vi "Periodic Tasks.vi"(8 "error in (no error)":errorcluster) -> ()   [LabVIEW 2015]
doc: "This VI runs in parallel to other tasks. It can contain as many user-defined periodic loops as you need. These can carry out PID or other sorts of timed response."
uses:
  arm/arm.lvclass/arm.ctl
  Robot Global Data.vi
  <vilib>/addons/control/pid/pid.llb/PID (DBL).vi
  <vilib>/Rock Robotics/Network Tables/NT Read Number.vi
  <vilib>/Rock Robotics/Network Tables/NT Write Number.vi
  <vilib>/Rock Robotics/WPI/RobotDrive/WPI_RobotDriveArcadeDrive_Standard(NoSaturation).vi
  <vilib>/addons/control/pid/NI_PID_pid.lvlib
  <vilib>/Analysis/NI_AALPro.lvlib
  shooter/shooter.lvclass
  <vilib>/Analysis/coordinate.llb/2D Cartesian Coordinate Shift (Scalar).vi
  <vilib>/Rock Robotics/Network Tables/NT Read String.vi
  <vilib>/Analysis/coordinate.llb/2D Cartesian Coordinate Shift (Array).vi
  intake/intake.lvclass
  arm/arm.lvclass
  drive/drive.lvclass
  <vilib>/Analysis/coordinate.llb/2D Cartesian Coordinate Rotation (Scalar).vi
panel:
  out "Waveform Chart":dbl(graph)
  out "CDF Arm Down":bool
  out "error out (no error)":errorcluster
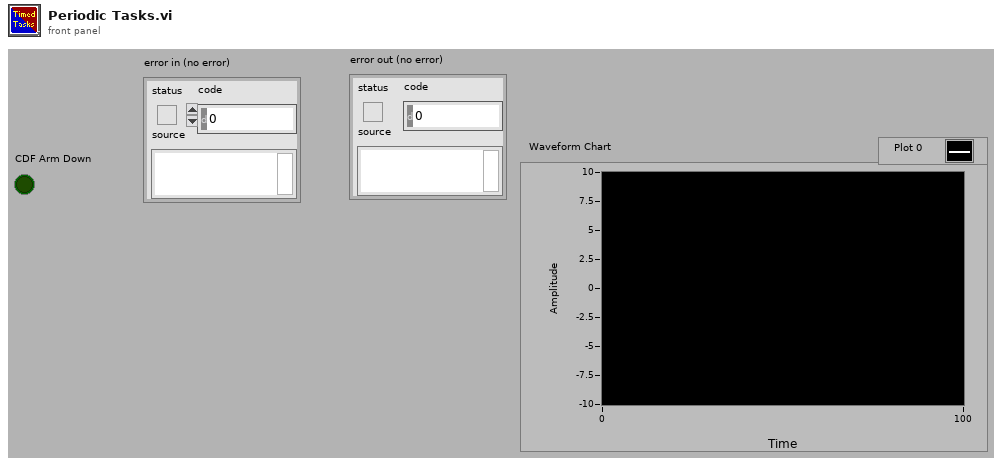
[diagram p1: front panel]
types:
  T1 = cluster{"theta":dbl, "x":dbl, "y":dbl, "xServo":dbl, "yServo":dbl}
  T2 = typedef "WPI_PotentiometerDevRef.ctl" = cluster{"DevStatus":errorcluster, "Analog Channel":T3, "Invert Output":bool}
  T3 = typedef "FPGA_AIChannel.ctl" = enum8{"AI 0", "AI 1", "AI 2", "AI 3", "AI MXP 0", "AI MXP 1", "AI MXP 2", "AI MXP 3", "Invalid"}
  T4 = typedef "WPI_ServoDeviceRef.ctl" = cluster{"DeviceStatus":errorcluster, "PWM Channel":T5, "DeadBand":T6}
  T5 = typedef "FPGA_DIOPWMChannel.ctl" = enum8{"PWM 0", "PWM 1", "PWM 2", "PWM 3", "PWM 4", "PWM 5", "PWM 6", "PWM 7", "PWM 8", "PWM 9", "PWM MXP 0", "PWM MXP 1", "PWM MXP 2", "PWM MXP 3", "PWM MXP 4", "PWM MXP 5", "PWM MXP 6", "PWM MXP 7", "PWM MXP 8", "PWM MXP 9", "Invalid"}
  T6 = typedef "WPI_PWMDeadband.ctl" = cluster{"Name":string, "maxPositivePwm":i32, "minPositivePwm":i32, "centerPwm":i32, "maxNegativePwm":i32, "minNegativePwm":i32, "angularRange":u16}
  T7 = typedef "WPI_GyroDevRef.ctl" = cluster{"DevStatus":errorcluster, "Analog Channel":T3, "Offset":dbl, "Gain (VoltsPerDegree/Second)":dbl, "Gyro Type":enum16{"Analog", "XRS450"}, "Handle":i32, "SPI Bus":T8, "Device Found":bool, "Sample Rate":dbl, "Calibrate On Open":bool}
  T8 = typedef "spi_bus.ctl" = enum16{"SPI On-Board, CS0", "SPI On-Board, CS1", "SPI On-Board, CS2", "SPI On-Board, CS3", "SPI MXP", "Invalid"}
  T9 = cluster{"theta":dbl, "x":dbl, "y":dbl, "xServo":dbl, "yServo":dbl}[]
  T10 = cluster{"proportional gain (Kc)":dbl, "integral time (Ti, min)":dbl, "derivative time (Td, min)":dbl}
  T11 = typedef "WPI_MotorControlDeviceRef.ctl" = cluster{"DeviceStatus":errorcluster, "Type":T12, "PWM":cluster{"PWM Channel":T5, "DeadBand":T6}, "CAN":cluster{"Device Number":u8, "Control Mode":T13, "Semaphore":T14, "Max Vout":dbl, "TalonSRX Control Mode":T15}, "Invert":bool}
  T12 = typedef "WPI_MotorControlType.ctl" = enum16{"PWM", "CAN", "CANTalonSRX"}
  T13 = typedef "WPI_CANJaguar_ControlMode.ctl" = enum8{"Percent VBus", "Current", "Speed", "Position", "Voltage"}
  T14 = typedef "Semaphore RefNum" = refnum<k1>
  T15 = typedef "WPI_CANTalonSRX_APIControlMode.ctl" = enum8{"Percent VBus", "Speed", "Position", "Slave", "Unchanged / Invalid", "Voltage Compensation", "Current", "Motion Profile"}
  T16 = typedef "WPI_AccelerometerDevRef.ctl" = cluster{"DevStatus":errorcluster, "Scaling":T17, "Analog Channels":T18, "I2C Bus":T19, "SPI Bus":T8, "Accel Range":T20, "ADXL Axes":T21, "Handle":i32, "Device Address":u8, "Accel Type":enum16{"Analog", "ADXL345 I2C", "ADXL345 SPI", "Internal", "ADXL362 SPI"}}
  T17 = typedef "WPI_AccelerometerScaling.ctl" = cluster{"Gain (VoltsPerG)":dbl, "Center Voltage":dbl}
  T18 = typedef "WPI_AccelerometerAnalogChannels.ctl" = cluster{"X-Axis":T3, "Y-Axis":T3, "Z-Axis":T3}
  T19 = typedef "i2c_bus.ctl" = enum16{"I2C On-Board", "I2C MXP", "Invalid"}
  T20 = typedef "ADXL345 Range.ctl" = u8
  T21 = typedef "WPI_AccelerometerADXL345 Axes.ctl" = cluster{"X-Axis":bool, "Y-Axis":bool, "Z-Axis":bool}
  T22 = cluster{"X-Axis":dbl, "Y-Axis":dbl, "Z-Axis":dbl}
  T23 = typedef "WPI_RobotDriveDevRef.ctl" = cluster{"DevStatus":errorcluster, "Motors[]":T11[], "Square Inputs":bool, "Max Output":dbl}
  T24 = enum16{"open", "replace", "create", "open or create", "replace or create", "replace or create with confirmation"}
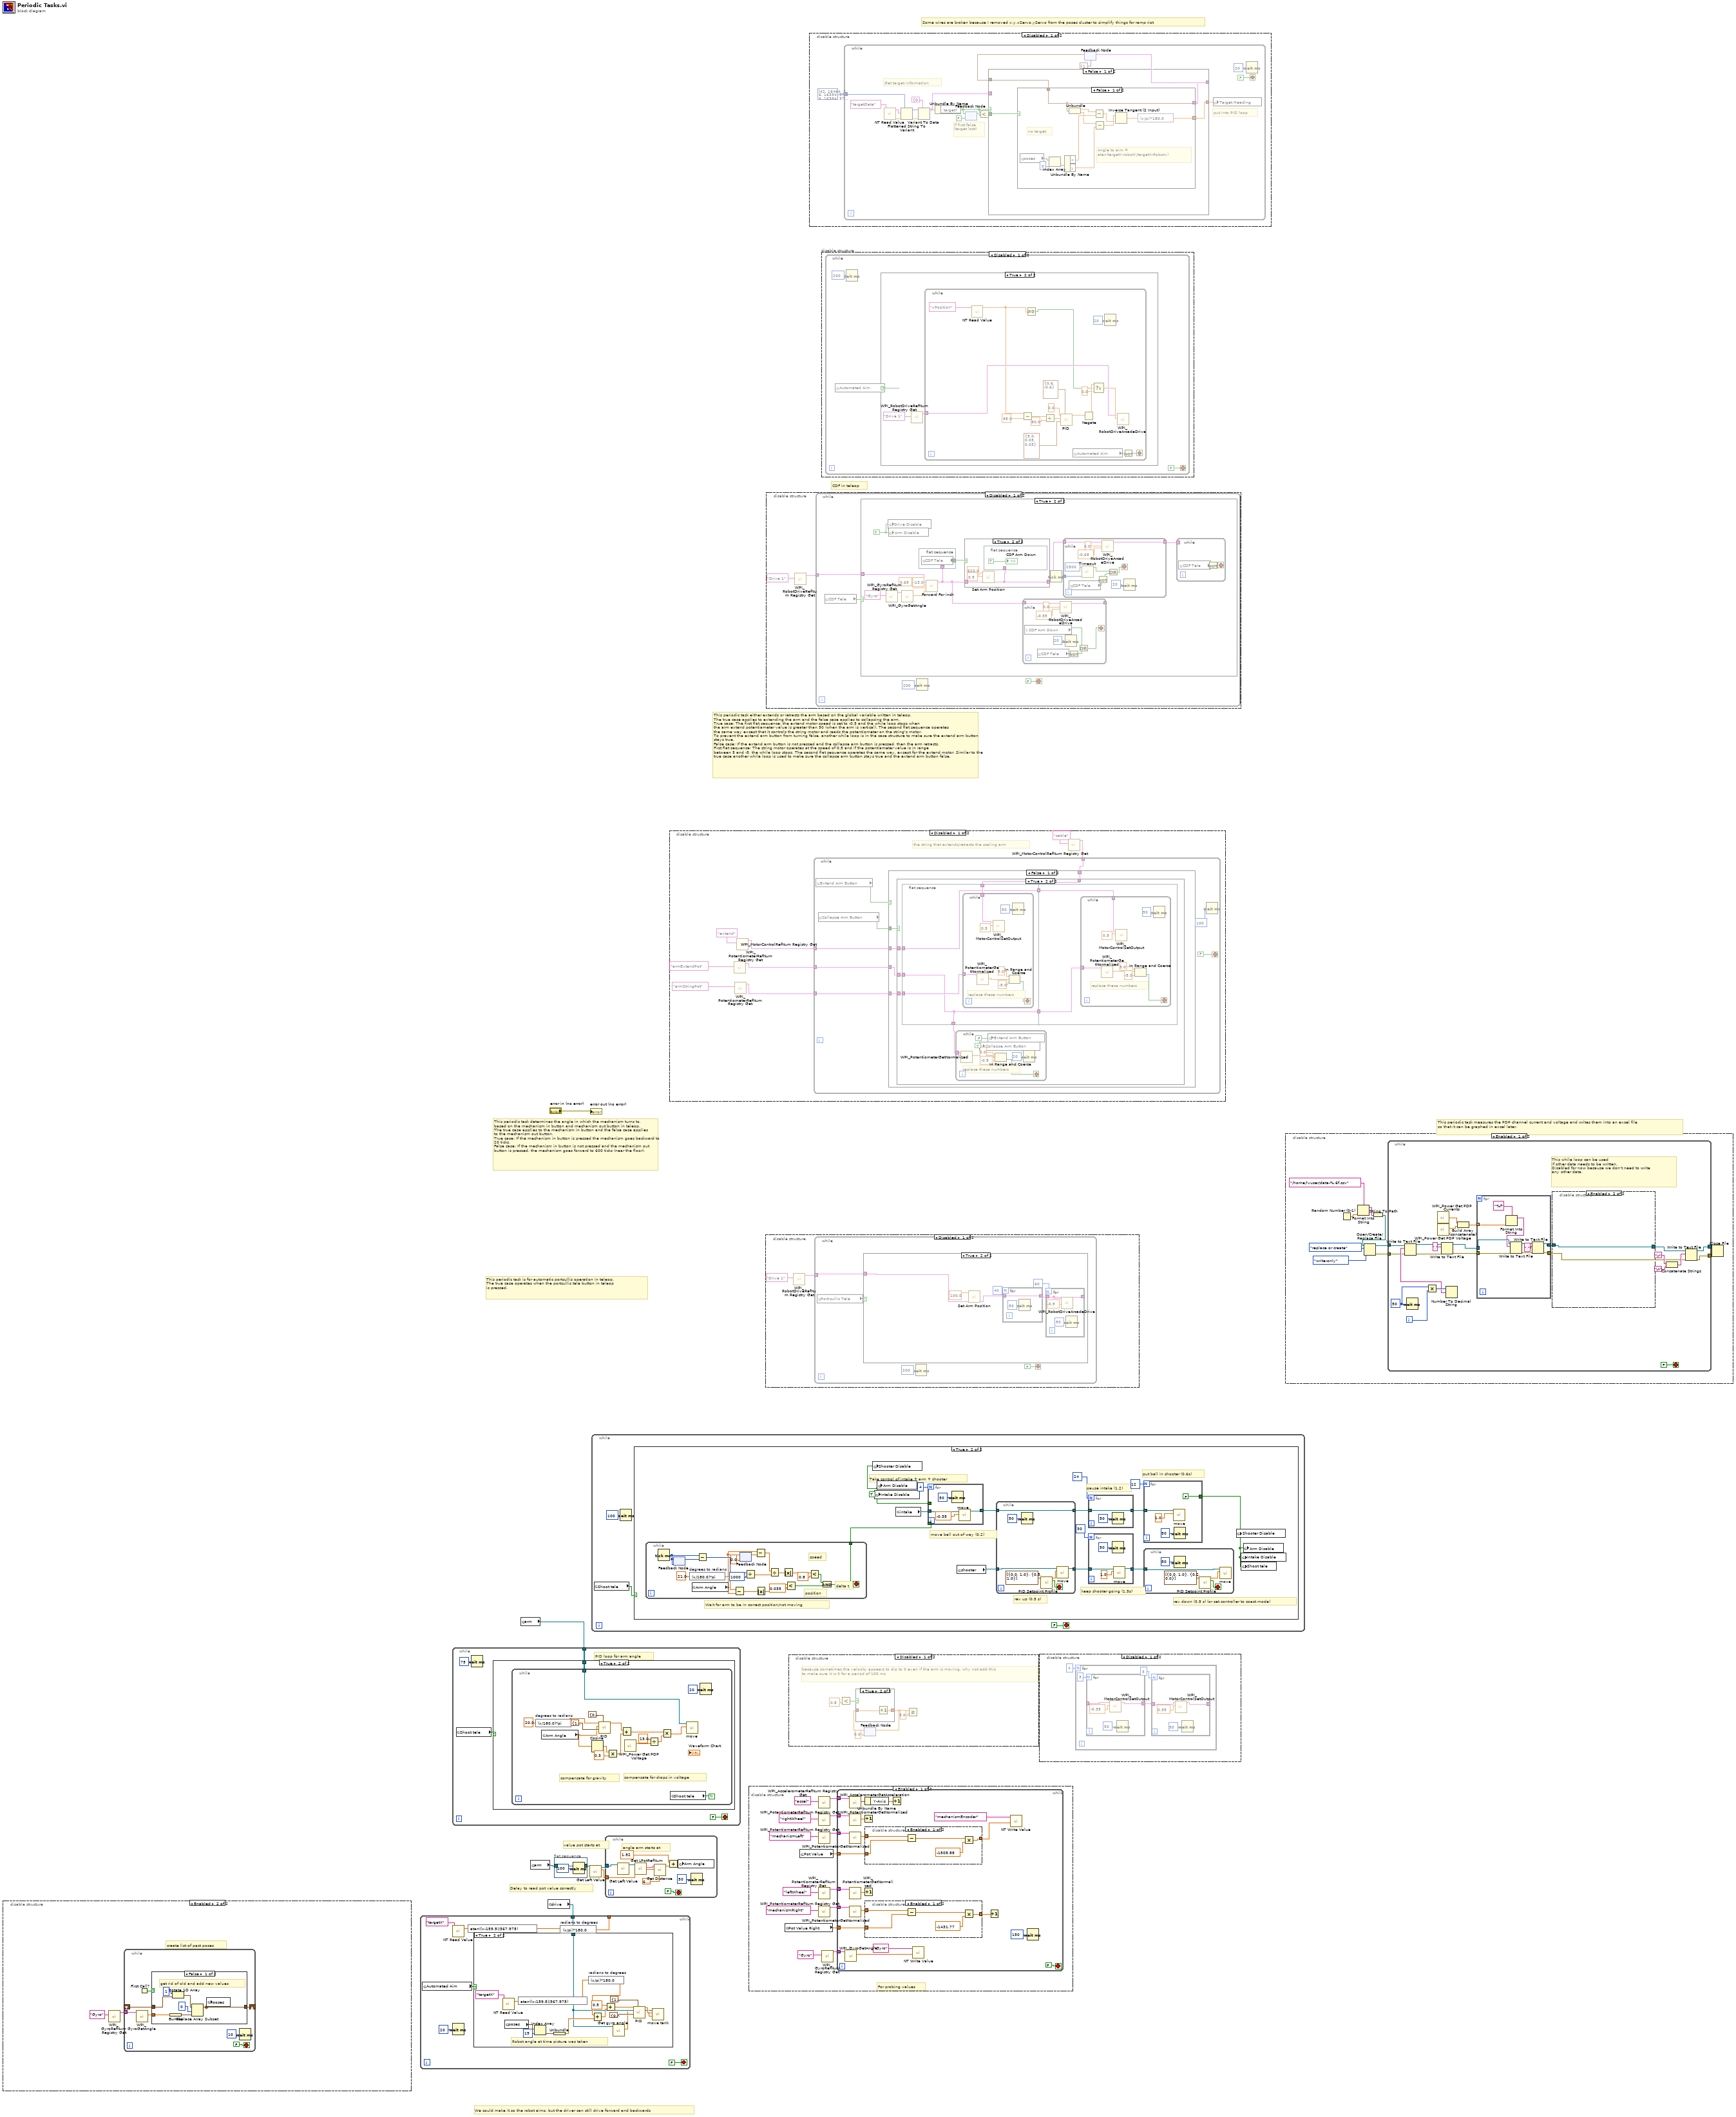
[diagram p0: block diagram]
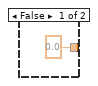
[diagram p4: hidden frame]
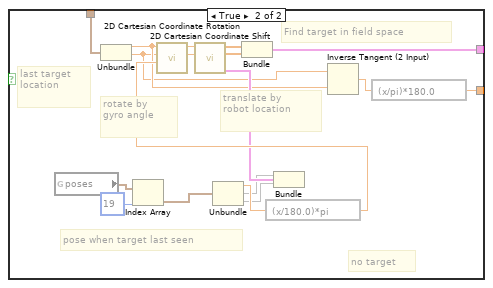
[diagram p8: hidden frame]
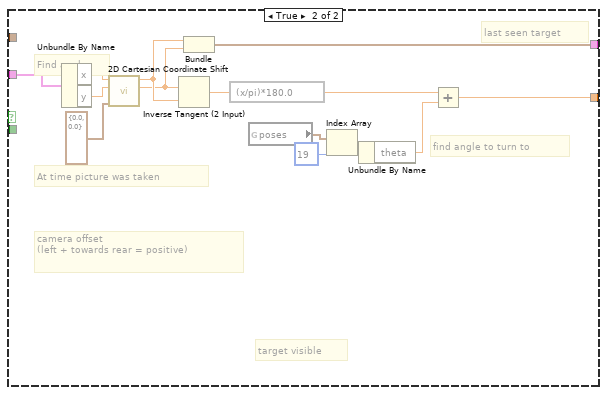
[diagram p9: hidden frame]
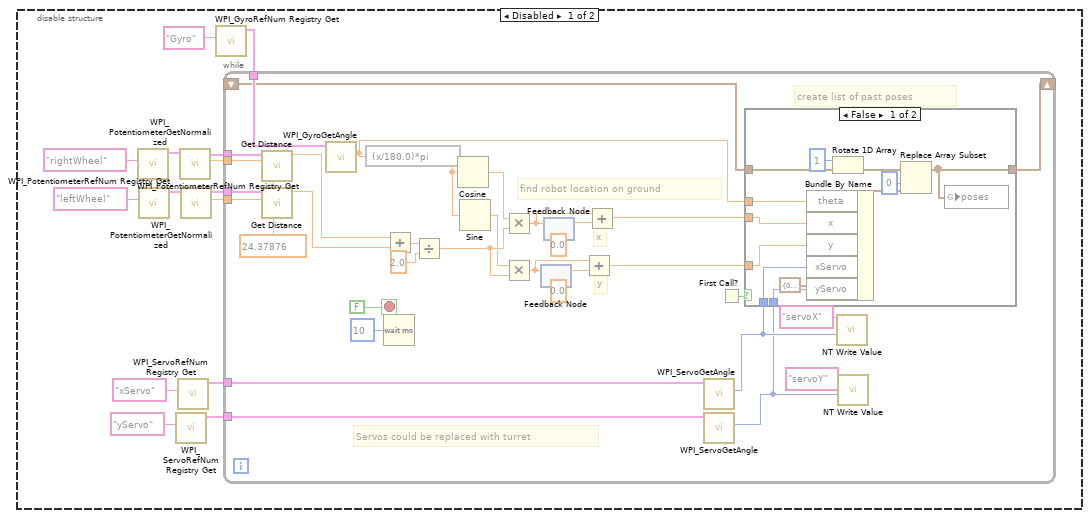
[diagram p11: hidden frame]
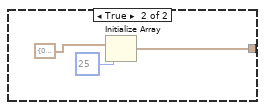
[diagram p12: hidden frame]
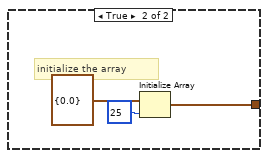
[diagram p13: hidden frame]
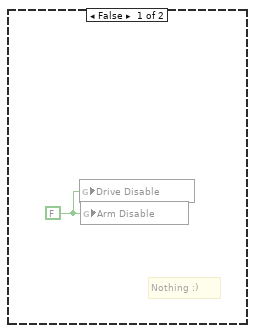
[diagram p16: hidden frame]
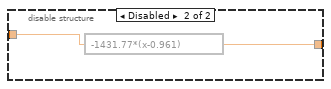
[diagram p19: hidden frame]
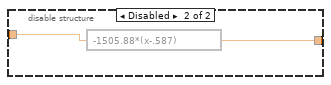
[diagram p20: hidden frame]
diagram:
  # "We could make it so the robot aims, but the driver can still drive forward and backwards"
  # "Delay to read pot value correctly"
  # "Some wires are broken because I removed x,y,xServo,yServo from the poses cluster to simplify things for ramp riot"
  # "value pot starts at"
  # "CDF in teleop"
  # "This periodic task either extends or retracts the arm based on the global variable written in teleop.\nThe true case applies to extending the arm and the false case applies to collapsing the arm. \nTrue case: The first flat sequence: the extend motor speed is set to -0.5 and the while loop stops when\nthe arm extend potentiameter value is greater than 90 (when the arm is vertical). The second flat sequence operates\nthe same way except that it controls the string motor and reads the potentiometer on the string's motor. \nTo prevent the extend arm button from turning false, another while loop is in the case structure to make sure the extend arm button \nstays true. \nFalse case: If the extend arm button is not pressed and the collapse arm button is pressed, then the arm retracts.\nFirst flat sequence: The string motor operates at the speed of 0.5 and if the potentiameter value is in range \nbetween 5 and -5, the while loop stops. The second flat sequence operates the same way, except for the extend motor. Similar to the \ntrue case another while loop is used to make sure the collapse arm button stays true and the extend arm button false."
  # "This periodic task measures the PDP channel current and voltage and writes them into an excel file \nso that it can be graphed in excel later."
  # "This periodic task is for automatic portcullis operation in teleop. \nThe true case operates when the portcullis tele button in teleop \nis pressed."
  # "This periodic task determines the angle in which the mechanism turns to, \nbased on the mechanism in button and mechanism out button in teleop.\nThe true case applies to the mechanism in button and the false case applies\nto the mechanism out button. \nTrue case: If the mechanism in button is pressed the mechanism goes backward to\n20 ticks. \nFalse case: If the mechanism in button is not pressed and the mechanism out\nbutton is pressed, the mechanism goes forward to 600 ticks (near the floor)."
  n1 = disable-structure shown="Enabled" {
    frame Disabled {
      n2 = call <vilib>:"WPI_PotentiometerRefNum Registry Get.vi"("refnum name"="rightWheel") -> ("PotDevRef"=w21:T2)  [unwired: 9 in, 1 out]
      n3 = call <vilib>:"WPI_PotentiometerRefNum Registry Get.vi"("refnum name"="leftWheel") -> ("PotDevRef"=w19:T2)  [unwired: 9 in, 1 out]
      n4 = call <vilib>:"WPI_ServoRefNum Registry Get.vi"("refnum name"="yServo") -> ("ServoDeviceRef"=w8:T4)  [unwired: 9 in, 1 out]
      n5 = call <vilib>:"WPI_ServoRefNum Registry Get.vi"("refnum name"="xServo") -> ("ServoDeviceRef"=w9:T4)  [unwired: 9 in, 1 out]
      n6 = call <vilib>:"WPI_PotentiometerGetNormalized.vi"("PotDevRef"=w21) -> ("Normalized Value"=w13:dbl, "PotDevRef"=w16:T2)  [unwired: 8 in, 1 out]
      n7 = call <vilib>:"WPI_PotentiometerGetNormalized.vi"("PotDevRef"=w19) -> ("Normalized Value"=w14:dbl, "PotDevRef"=w15:T2)  [unwired: 8 in, 1 out]
      n8 = call <vilib>:"WPI_GyroRefNum Registry Get.vi"("refnum name"="Gyro") -> ("GyroDevRef"=w12:T7)  [unwired: 9 in, 1 out]
      n9 = while {
        tunnel: w16 -> [w54]
        tunnel: w15 -> [w53]
        tunnel: w14 -> [w52]
        tunnel: w13 -> [w51]
        tunnel: w12 -> [w34]
        shift-right: [w30] -> _
        shift-left: _ -> [w29]
        tunnel: w9 -> [w25]
        tunnel: w8 -> [w24]
        stop <- FALSE stop-if-true
        w50 = 24.37876 ("distance/rotation")
        # "Servos could be replaced with turret"
        # "create list of past poses"
        # "find robot location on ground"
        # "y"
        # "x"
        n10 = call "Get Distance.vi"("distance/rotation"=w50, "Starting value"=w51, "PotDevRef"=w54) -> ("Distance"=w36:dbl)  [unwired: 8 in]
        n11 = call "Get Distance.vi"("distance/rotation"=w50, "Starting value"=w52, "PotDevRef"=w53) -> ("Distance"=w35:dbl)  [unwired: 8 in]
        n12 = call <vilib>:"WPI_GyroGetAngle.vi"("GyroDevRef"=w34) -> ("Angle"=w28:dbl)  [unwired: 6 in, 4 out]
        n13 = expression code="(x/180.0)*pi" ("degrees to radians")(w28) -> (w45:dbl)
        n14 = Wait (ms)(milliseconds to wait=u32 10) -> ()  [unwired: 1 out]
        n15 = Add(x=w36, y=w35) -> (x+y=w48:dbl)
        n16 = Divide(x=w48, y=2.0) -> (x/y=w44:dbl)
        n17 = Cosine(x=w45) -> (cos(x)=w46:dbl)
        n18 = Sine(x=w45) -> (sin(x)=w43:dbl)
        n19 = Multiply(x=w46, y=w44) -> (x*y=w41:dbl)
        n20 = Multiply(x=w43, y=w44) -> (x*y=w37:dbl)
        n21 = feedback #1(0.0) -> (w38:dbl)
        n22 = feedback-in #1(w37) -> ()
        n23 = feedback #2(0.0) -> (w42:dbl)
        n24 = feedback-in #2(w41) -> ()
        n25 = Add(x=w37, y=w38) -> (x+y=w27:dbl)
        n26 = Add(x=w41, y=w42) -> (x+y=w26:dbl)
        n27 = call <vilib>:"WPI_ServoGetAngle.vi"("ServoDeviceRef"=w25) -> ("Angle"=w23:u16)  [unwired: 7 in, 2 out]
        n28 = call <vilib>:"WPI_ServoGetAngle.vi"("ServoDeviceRef"=w24) -> ("Angle"=w22:u16)  [unwired: 7 in, 2 out]
        n29 = First Call?() -> (First Call?: T/F=w33:bool)
        n30 = case shown="False" w33 {
          tunnel: [w56 w69] -> w30
          tunnel: w29 -> [w67 _]
          tunnel: w28 -> [w63 _]
          tunnel: w26 -> [w59 _]
          tunnel: w27 -> [w60 _]
          tunnel: w23 -> [w58 _]
          tunnel: w22 -> [w57 _]
          frame False {
            n31 = Bundle By Name(cluster=T1 {"theta"=0.0, "x"=0.0, "y"=0.0, "xServo"=0.0, "yServo"=0.0}, "theta"=w63, "x"=w59, "y"=w60, "xServo"=w58, "yServo"=w57) -> (w61:T1)
            n32 = Rotate 1D Array(1:w67, 2:1 ("n")) -> (0:w65:T9)
            n33 = Replace Array Subset(array=w65, new element=w61, index=0) -> (w56:T9)
            n34 = global write "Robot Global Data.vi" "poses"(w56) -> ()
          }
          frame True {
            n35 = Initialize Array(T1 {"theta"=0.0, "x"=0.0, "y"=0.0, "xServo"=0.0, "yServo"=0.0}, 25 ("dimension size")) -> (w69:T9)
          }
        }
        n36 = call-poly <vilib>:"NT Write Value.vi"("Numeric"=w23, "Name"="servoX") -> ()  [unwired: 9 in, 1 out]
        n37 = call-poly <vilib>:"NT Write Value.vi"("Numeric"=w22, "Name"="servoY") -> ()  [unwired: 9 in, 1 out]
      }
    }
    frame Enabled {
      # "create list of past poses"
      n38 = call <vilib>:"WPI_GyroRefNum Registry Get.vi"("refnum name"="Gyro") -> ("GyroDevRef"=w71:T7)  [unwired: 9 in, 1 out]
      n39 = while {
        tunnel: w71 -> [w77]
        shift-right: [w75] -> _
        shift-left: _ -> [w74]
        stop <- FALSE stop-if-true
        n40 = call <vilib>:"WPI_GyroGetAngle.vi"("GyroDevRef"=w77) -> ("Angle"=w73:dbl)  [unwired: 6 in, 4 out]
        n41 = First Call?() -> (First Call?: T/F=w76:bool)
        n42 = case shown="False" w76 {
          tunnel: [w82 w88] -> w75
          tunnel: w74 -> [w86 _]
          tunnel: w73 -> [w81 _]
          frame False {
            # "get rid of old and add new values"
            n43 = Bundle("Angle"=w81) -> (w80:cluster{"Angle":dbl})  [unwired: 1 in]
            n44 = Rotate 1D Array(1:w86, 2:1 ("n")) -> (0:w84:cluster{"theta":dbl}[])
            n45 = Replace Array Subset(array=w84, new element=w80, index=0) -> (w82:cluster{"theta":dbl}[])
            n46 = global write "Robot Global Data.vi" "poses"(w82) -> ()
          }
          frame True {
            # "initialize the array"
            n47 = Initialize Array(cluster{"theta":dbl} {"theta"=0.0}, 25 ("dimension size")) -> (w88:cluster{"theta":dbl}[])
          }
        }
        n48 = Wait (ms)(milliseconds to wait=u32 10) -> ()  [unwired: 1 out]
      }
    }
  }
  n49 = global read "Robot Global Data.vi" "arm"() -> (w2:refnum<class "arm.lvclass">)
  n50 = while {
    tunnel: w2 -> [w90]
    stop <- FALSE stop-if-true
    # "PID loop for arm angle"
    n51 = global read "Robot Global Data.vi" "Shoot tele"() -> (w93:bool)
    n52 = Wait (ms)(milliseconds to wait=u32 75) -> ()  [unwired: 1 out]
    n53 = case shown="True" w93 {
      tunnel: w90 -> [_ w94]
      frame False {
      }
      frame True {
        n54 = while {
          tunnel: w94 -> [w95]
          stop <- w110 continue-if-true
          # "compensate for drops in voltage"
          # "compensate for gravity"
          n55 = expression code="(x/180.0)*pi" "degrees to radians"(20.0 ("angle B 2")) -> (w106:dbl)
          n56 = global read "Robot Global Data.vi" "Arm Angle"() -> (w98:dbl)
          n57 = Cosine(x=w98) -> (cos(x)=w104:dbl)
          n58 = call-poly <vilib>:"PID.vi"("output range"=cluster{"output high":dbl, "output low":dbl} {"output high"=0.7, "output low"=-0.7}, "PID gains"=T10 {"proportional gain (Kc)"=1.1, "integral time (Ti, min)"=0.008, "derivative time (Td, min)"=0.0001} ("PID arm gains"), "process variable"=w98, "setpoint"=w106) -> ("output"=w103:dbl)  [unwired: 6 in, 1 out]
          n59 = Multiply(x=w104, y=0.3) -> (x*y=w102:dbl)
          n60 = Add(x=w103, y=w102) -> (x+y=w99:dbl)
          n61 = call <vilib>:"WPI_Power Get PDP Voltage.vi"() -> ("voltage (V)"=w100:dbl)  [unwired: 14 in, 1 out]
          n62 = Divide(x=13.0, y=w100) -> (x/y=w97:dbl)
          n63 = Multiply(x=w99, y=w97) -> (x*y=w96:dbl)
          n64 = global read "Robot Global Data.vi" "Shoot tele"() -> (w110:bool)
          n65 = call "move.vi"("Speed"=w96, "arm.lvclass"=w95) -> ()  [unwired: 9 in, 1 out]
          n66 = Wait (ms)(milliseconds to wait=u32 20) -> ()  [unwired: 1 out]
        }
      }
    }
  }
  n67 = global read "Robot Global Data.vi" "arm"() -> (w3:refnum<class "arm.lvclass">)
  n68 = global read "Robot Global Data.vi" "drive"() -> (w1:refnum<class "drive.lvclass">)
  n69 = while {
    tunnel: w1 -> [w116]
    tunnel: [w112] -> _
    stop <- FALSE stop-if-true
    n70 = global read "Robot Global Data.vi" "Automated Aim"() -> (w117:bool)
    n71 = call-poly <vilib>:"NT Read Value.vi"("Name"="targetX") -> ("Numeric"=w115:dbl)  [unwired: 9 in, 1 out]
    n72 = Wait (ms)(milliseconds to wait=u32 20) -> ()  [unwired: 1 out]
    n73 = expression code="atan((x-159.5)/367.975)"(w115) -> (w113:dbl)
    n74 = case shown="True" w117 {
      tunnel: w116 -> [_ w121]
      frame False {
      }
      frame True {
        # "Robot angle at time picture was taken"
        n75 = call-poly <vilib>:"NT Read Value.vi"("Name"="targetX") -> ("Numeric"=w134:dbl)  [unwired: 9 in, 1 out]
        n76 = global read "Robot Global Data.vi" "poses"() -> (w133:cluster{"theta":dbl}[])
        n77 = expression code="atan((x-159.5)/367.975)"(w134) -> (w129:dbl)
        n78 = Index Array(array=w133, index=19) -> (element=w131:cluster{"theta":dbl})
        n79 = Unbundle(w131) -> ("theta"=w130:dbl)
        n80 = expression code="(x/pi)*180.0" "radians to degrees"(w129) -> (w128:dbl)
        n81 = Add(x=w128, y=w130) -> (x+y=w125:dbl)
        n82 = Add(x=0.5, y=w125) -> (x+y=w123:dbl)
        n83 = call "Get gyro angle.vi"("drive in"=w121) -> ("Angle"=w120:dbl)  [unwired: 9 in, 1 out]
        n84 = call-poly <vilib>:"PID.vi"("output range"=cluster{"output high":dbl, "output low":dbl} {"output high"=1.0, "output low"=-1.0}, "PID gains"=T10 {"proportional gain (Kc)"=0.07, "integral time (Ti, min)"=0.004, "derivative time (Td, min)"=1e-05} ("PID turn angle gains"), "process variable"=w120, "setpoint"=w123) -> ("output"=w122:dbl)  [unwired: 6 in, 1 out]
        n85 = call "move tank.vi"("Right Value"=w122, "Left Value"=w122, "drive.lvclass"=w121) -> ()  [unwired: 8 in, 1 out]
      }
    }
    n86 = expression code="(x/pi)*180.0" "radians to degrees"(w113) -> (w112:dbl)
  }
  n87 = flat-sequence {
    tunnel: w3 -> [w137]
    tunnel: [w137] -> w6
    frame #0 {
      n88 = Wait (ms)(milliseconds to wait=u32 100) -> ()  [unwired: 1 out]
    }
  }
  n89 = call "Get Left Value.vi"("arm.lvclass"=w6) -> ("Value"=w5:dbl, "arm.lvclass"=w4:refnum<class "arm.lvclass">)  [unwired: 9 in]
  n90 = while {
    stop <- FALSE stop-if-true
    n91 = global read "Robot Global Data.vi" "Shoot tele"() -> (w138:bool)
    n92 = Wait (ms)(milliseconds to wait=u32 100) -> ()  [unwired: 1 out]
    n93 = case shown="True" w138 {
      frame False {
      }
      frame True {
        w144 = TRUE ("Intake Disable")
        # "Wait for arm to be in correct position/not moving"
        # "Take control of intake + arm + shooter"
        # "put ball in shooter (0.6s)"
        # "pause intake (1.2)"
        # "rev down (0.5 s) (or set controller to coast mode)"
        # "keep shooter going (1.5s)"
        # "rev up (0.5 s)"
        # "move ball out of way (0.2)"
        n94 = while {
          tunnel: [w155] -> w147
          stop <- w155 stop-if-true
          # "position"
          # "speed"
          # "delta t"
          n95 = Tick Count (ms)() -> (millisecond timer value=w168:u32)
          n96 = feedback #3(w168) -> (w167:u32)
          n97 = feedback-in #3(w168) -> ()
          n98 = expression code="(x/180.0)*pi" "degrees to radians"(21.0 ("angle B 2")) -> (w162:dbl)
          n99 = global read "Robot Global Data.vi" "Arm Angle"() -> (w161:dbl)
          n100 = Subtract(x=w168, y=w167) -> (x-y=w169:u32)
          n101 = Subtract(x=w162, y=w161) -> (x-y=w157:dbl)
          n102 = feedback #4(0.0 ("Arm Angle")) -> (w171:dbl)
          n103 = feedback-in #4(w161) -> ()
          n104 = Divide(x=w169, y=u32 1000) -> (x/y=w174:dbl)
          n105 = Subtract(x=w161, y=w171) -> (x-y=w173:dbl)
          n106 = Absolute Value(x=w157) -> (abs(x)=w156:dbl)
          n107 = Divide(x=w173, y=w174) -> (x/y=w166:dbl)
          n108 = Absolute Value(x=w166) -> (abs(x)=w163:dbl)
          n109 = Less?(x=w156, y=0.035) -> (x < y?=w159:bool)
          n110 = Less?(x=w163, y=0.8) -> (x < y?=w164:bool)
          n111 = And(x=w164, y=w159) -> (x .and. y?=w155:bool)
        }
        n112 = global write "Robot Global Data.vi" "Shooter Disable"(w144) -> ()
        n113 = global write "Robot Global Data.vi" "Intake Disable"(w144) -> ()
        n114 = global write "Robot Global Data.vi" "Arm Disable"(w144) -> ()
        n115 = global read "Robot Global Data.vi" "intake"() -> (w141:refnum<class "intake.lvclass">)
        n116 = for {
          N: 4 -> [_]
          tunnel: [w190] -> w145
          tunnel: w144 -> [_]
          tunnel: w147 -> [_]
          tunnel: w141 -> [w191]
          n117 = Wait (ms)(milliseconds to wait=u32 50) -> ()  [unwired: 1 out]
          n118 = call "move.vi"("Speed"=-0.35 ("Left axis value"), "intake.lvclass"=w191) -> ("intake.lvclass"=w190:refnum<class "intake.lvclass">)  [unwired: 9 in]
        }
        n119 = global read "Robot Global Data.vi" "shooter"() -> (w142:refnum<class "shooter.lvclass">)
        n120 = while {
          tunnel: w142 -> [w196]
          tunnel: [w194] -> w153
          tunnel: [w197] -> w146
          tunnel: w145 -> [w197]
          stop <- w200 stop-if-true
          n121 = Wait (ms)(milliseconds to wait=u32 50) -> ()  [unwired: 1 out]
          n122 = call <vilib>:"PID Setpoint Profile.vi"("setpoint profile"=cluster{"time (s)":dbl, "setpoint":dbl}[] [{"time (s)"=0.0, "setpoint"=1.0}, {"time (s)"=0.5, "setpoint"=1.0}]) -> ("profile complete?"=w200:bool, "setpoint"=w195:dbl)  [unwired: 5 in, 2 out]
          n123 = call "move.vi"("Speed"=w195, "shooter.lvclass"=w196) -> ("shooter.lvclass"=w194:refnum<class "shooter.lvclass">)  [unwired: 9 in]
        }
        n124 = for {
          N: 24 -> [_]
          tunnel: [w184] -> w150
          tunnel: w146 -> [w184]
          n125 = Wait (ms)(milliseconds to wait=u32 50) -> ()  [unwired: 1 out]
        }
        n126 = for {
          N: 30 -> [_]
          tunnel: w153 -> [w188]
          tunnel: [w187] -> w148
          n127 = Wait (ms)(milliseconds to wait=u32 50) -> ()  [unwired: 1 out]
          n128 = call "move.vi"("Speed"=1.0 ("Left axis value"), "shooter.lvclass"=w188) -> ("shooter.lvclass"=w187:refnum<class "shooter.lvclass">)  [unwired: 9 in]
        }
        n129 = for {
          N: 12 -> [_]
          tunnel: w150 -> [w181]
          tunnel: [FALSE ("Shoot tele")] -> w143
          n130 = call "move.vi"("Speed"=1.0 ("Left axis value"), "intake.lvclass"=w181) -> ()  [unwired: 9 in, 1 out]
          n131 = Wait (ms)(milliseconds to wait=u32 50) -> ()  [unwired: 1 out]
        }
        n132 = while {
          tunnel: w148 -> [w176]
          stop <- w178 stop-if-true
          n133 = Wait (ms)(milliseconds to wait=u32 50) -> ()  [unwired: 1 out]
          n134 = call <vilib>:"PID Setpoint Profile.vi"("setpoint profile"=cluster{"time (s)":dbl, "setpoint":dbl}[] [{"time (s)"=0.0, "setpoint"=1.0}, {"time (s)"=0.2, "setpoint"=0.0}]) -> ("profile complete?"=w178:bool, "setpoint"=w175:dbl)  [unwired: 5 in, 2 out]
          n135 = call "move.vi"("Speed"=w175, "shooter.lvclass"=w176) -> ()  [unwired: 9 in, 1 out]
        }
        n136 = global write "Robot Global Data.vi" "Shooter Disable"(w143) -> ()
        n137 = global write "Robot Global Data.vi" "Intake Disable"(w143) -> ()
        n138 = global write "Robot Global Data.vi" "Shoot tele"(w143) -> ()
        n139 = global write "Robot Global Data.vi" "Arm Disable"(w143) -> ()
      }
    }
  }
  n140 = while {
    tunnel: w4 -> [w203]
    tunnel: w5 -> [w207]
    stop <- FALSE stop-if-true
    # "angle arm starts at"
    n141 = call "Get Left Value.vi"("arm.lvclass"=w203) -> ("arm.lvclass"=w202:refnum<class "arm.lvclass">)  [unwired: 9 in, 1 out]
    n142 = call "Get LPotRefNum.vi"("arm in"=w202) -> ("PotDevRef"=w201:T2)  [unwired: 9 in, 1 out]
    n143 = call "Get Distance.vi"("distance/rotation"=6.283185307179586, "Starting value"=w207, "PotDevRef"=w201) -> ("Distance"=w206:dbl)  [unwired: 8 in]
    n144 = Add(x=1.92 ("Starting value"), y=w206) -> (x+y=w205:dbl)
    n145 = global write "Robot Global Data.vi" "Arm Angle"(w205) -> ()
    n146 = Wait (ms)(milliseconds to wait=u32 50) -> ()  [unwired: 1 out]
  }
  n147 = disable-structure shown="Disabled" {
    frame Disabled {
      # "the string that extends/retracts the scaling arm"
      n148 = call <vilib>:"WPI_PotentiometerRefNum Registry Get.vi"("refnum name"="armExtendPot") -> ("PotDevRef"=w214:T2)  [unwired: 9 in, 1 out]
      n149 = call <vilib>:"WPI_PotentiometerRefNum Registry Get.vi"("refnum name"="armStringPot") -> ("PotDevRef"=w213:T2)  [unwired: 9 in, 1 out]
      n150 = call <vilib>:"WPI_MotorControlRefNum Registry Get.vi"("refnum name"="extend") -> ("MotorControlDevRef"=w212:T11)  [unwired: 9 in, 1 out]
      n151 = call <vilib>:"WPI_MotorControlRefNum Registry Get.vi"("refnum name"="cable") -> ("MotorControlDevRef"=w211:T11)  [unwired: 9 in, 1 out]
      n152 = while {
        tunnel: w214 -> [w225]
        tunnel: w213 -> [w224]
        tunnel: w212 -> [w222]
        tunnel: w211 -> [w221]
        stop <- FALSE stop-if-true
        n153 = global read "Robot Global Data.vi" "Extend Arm Button"() -> (w220:bool)
        n154 = global read "Robot Global Data.vi" "Collapse Arm Button"() -> (w219:bool)
        n155 = case shown="False" w220 {
          tunnel: w219 -> [w231 _]
          tunnel: w225 -> [w230 w274]
          tunnel: w224 -> [w229 w272]
          tunnel: w222 -> [w227 w271]
          tunnel: w221 -> [w228 w270]
          frame False {
            n156 = case shown="True" w231 {
              tunnel: w230 -> [_ w238]
              tunnel: w229 -> [_ w237]
              tunnel: w228 -> [_ w236]
              tunnel: w227 -> [_ w234]
              frame False {
                # "Nothing :)"
              }
              frame True {
                n157 = flat-sequence {
                  tunnel: w238 -> [w247]
                  tunnel: w237 -> [w248]
                  tunnel: w236 -> [w250]
                  tunnel: [w249] -> w235
                  tunnel: w234 -> [w249]
                  tunnel: [w247] -> w233
                  tunnel: [w247] -> w232
                  tunnel: w235 -> [w260]
                  tunnel: w233 -> [w259]
                  frame #0 {
                    n158 = while {
                      tunnel: w250 -> [w257]
                      tunnel: w248 -> [w256]
                      stop <- w251 stop-if-true
                      # "replace these numbers"
                      n159 = call <vilib>:"WPI_PotentiometerGetNormalized.vi"("PotDevRef"=w256) -> ("Normalized Value"=w254:dbl)  [unwired: 8 in, 2 out]
                      n160 = call <vilib>:"WPI_MotorControlSetOutput.vi"("Output"=0.5, "MotorControlDevRef"=w257) -> ()  [unwired: 7 in, 3 out]
                      n161 = In Range and Coerce(upper limit=5.0, x=w254, lower limit=-5.0) -> (In Range?=w251:bool)  [unwired: 1 out]
                      n162 = Wait (ms)(milliseconds to wait=u32 50) -> ()  [unwired: 1 out]
                    }
                  }
                  frame #1 {
                    n163 = while {
                      tunnel: w260 -> [w267]
                      tunnel: w259 -> [w266]
                      stop <- w264 stop-if-true
                      # "replace these numbers"
                      n164 = call <vilib>:"WPI_PotentiometerGetNormalized.vi"("PotDevRef"=w266) -> ("Normalized Value"=w262:dbl)  [unwired: 8 in, 2 out]
                      n165 = call <vilib>:"WPI_MotorControlSetOutput.vi"("Output"=0.5, "MotorControlDevRef"=w267) -> ()  [unwired: 7 in, 3 out]
                      n166 = In Range and Coerce(upper limit=5.0 ("y"), x=w262, lower limit=-5.0) -> (In Range?=w264:bool)  [unwired: 1 out]
                      n167 = Wait (ms)(milliseconds to wait=u32 50) -> ()  [unwired: 1 out]
                    }
                  }
                }
                n168 = while {
                  tunnel: w232 -> [w246]
                  stop <- w239 stop-if-true
                  # "Extend"
                  # "replace these numbers"
                  n169 = call <vilib>:"WPI_PotentiometerGetNormalized.vi"("PotDevRef"=w246) -> ("Normalized Value"=w240:dbl)  [unwired: 8 in, 2 out]
                  n170 = global write "Robot Global Data.vi" "Collapse Arm Button"(TRUE ("Collapse Arm Button")) -> ()
                  n171 = global write "Robot Global Data.vi" "Extend Arm Button"(FALSE) -> ()
                  n172 = In Range and Coerce(upper limit=0.0 ("y"), x=w240, lower limit=-0.5) -> (In Range?=w239:bool)  [unwired: 1 out]
                  n173 = Wait (ms)(milliseconds to wait=u32 20) -> ()  [unwired: 1 out]
                }
              }
            }
          }
          frame True {
            n174 = flat-sequence {
              tunnel: w274 -> [w282]
              tunnel: [w280] -> w273
              tunnel: w272 -> [w280]
              tunnel: w271 -> [w281]
              tunnel: [w280] -> w269
              tunnel: w273 -> [w291]
              tunnel: w270 -> [w290]
              frame #0 {
                n175 = while {
                  tunnel: w282 -> [w288]
                  tunnel: w281 -> [w284]
                  stop <- w285 stop-if-true
                  # "replace these numbers"
                  n176 = call <vilib>:"WPI_PotentiometerGetNormalized.vi"("PotDevRef"=w288) -> ("Normalized Value"=w287:dbl)  [unwired: 8 in, 2 out]
                  n177 = call <vilib>:"WPI_MotorControlSetOutput.vi"("Output"=-0.5, "MotorControlDevRef"=w284) -> ()  [unwired: 7 in, 3 out]
                  n178 = Wait (ms)(milliseconds to wait=u32 40) -> ()  [unwired: 1 out]
                  n179 = Greater Or Equal?(x=w287, y=90.0) -> (x >= y?=w285:bool)
                }
              }
              frame #1 {
                n180 = while {
                  tunnel: w291 -> [w295]
                  tunnel: w290 -> [w293]
                  stop <- w294 stop-if-true
                  # "replace these numbers"
                  n181 = call <vilib>:"WPI_PotentiometerGetNormalized.vi"("PotDevRef"=w295) -> ("Normalized Value"=w297:dbl)  [unwired: 8 in, 2 out]
                  n182 = call <vilib>:"WPI_MotorControlSetOutput.vi"("Output"=-0.5, "MotorControlDevRef"=w293) -> ()  [unwired: 7 in, 3 out]
                  n183 = Greater Or Equal?(x=w297, y=90.0) -> (x >= y?=w294:bool)
                  n184 = Wait (ms)(milliseconds to wait=u32 40) -> ()  [unwired: 1 out]
                }
              }
            }
            n185 = while {
              tunnel: w269 -> [w276]
              stop <- w277 stop-if-true
              # "Extend"
              # "replace these numbers"
              n186 = call <vilib>:"WPI_PotentiometerGetNormalized.vi"("PotDevRef"=w276) -> ("Normalized Value"=w279:dbl)  [unwired: 8 in, 2 out]
              n187 = global write "Robot Global Data.vi" "Extend Arm Button"(TRUE) -> ()
              n188 = Greater Or Equal?(x=w279, y=90.0) -> (x >= y?=w277:bool)
            }
          }
        }
        n189 = Wait (ms)(milliseconds to wait=u32 100) -> ()  [unwired: 1 out]
      }
    }
    frame Enabled {
    }
  }
  n190 = disable-structure shown="Enabled" {
    frame Enabled {
      # "For probing values"
      n191 = global read "Robot Global Data.vi" "Pot Value Right"() -> (w305:dbl)
      n192 = global read "Robot Global Data.vi" "Pot Value"() -> (w306:dbl)
      n193 = call <vilib>:"WPI_AccelerometerRefNum Registry Get.vi"("refnum name"="accel") -> ("AccelerometerDevRef"=w310:T16)  [unwired: 9 in, 1 out]
      n194 = call <vilib>:"WPI_PotentiometerRefNum Registry Get.vi"("refnum name"="rightWheel") -> ("PotDevRef"=w303:T2)  [unwired: 9 in, 1 out]
      n195 = call <vilib>:"WPI_PotentiometerRefNum Registry Get.vi"("refnum name"="mechanismLeft") -> ("PotDevRef"=w301:T2)  [unwired: 9 in, 1 out]
      n196 = call <vilib>:"WPI_PotentiometerRefNum Registry Get.vi"("refnum name"="leftWheel") -> ("PotDevRef"=w302:T2)  [unwired: 9 in, 1 out]
      n197 = call <vilib>:"WPI_PotentiometerRefNum Registry Get.vi"("refnum name"="mechanismRight") -> ("PotDevRef"=w307:T2)  [unwired: 9 in, 1 out]
      n198 = call <vilib>:"WPI_GyroRefNum Registry Get.vi"("refnum name"="Gyro") -> ("GyroDevRef"=w299:T7)  [unwired: 9 in, 1 out]
      n199 = while {
        tunnel: w303 -> [w332]
        tunnel: w310 -> [w327]
        tunnel: w301 -> [w326]
        tunnel: w307 -> [w325]
        tunnel: w306 -> [w320]
        tunnel: w305 -> [w319]
        tunnel: w302 -> [w316]
        tunnel: w299 -> [w313]
        stop <- FALSE stop-if-true
        n200 = call <vilib>:"WPI_GyroGetAngle.vi"("GyroDevRef"=w313) -> ("Angle"=w314:dbl)  [unwired: 6 in, 4 out]
        n201 = call <vilib>:"WPI_AccelerometerGetAcceleration.vi"("AccelerometerDevRef"=w327) -> ("Accelerations"=w328:T22)  [unwired: 8 in, 2 out]
        n202 = call <vilib>:"WPI_PotentiometerGetNormalized.vi"("PotDevRef"=w332) -> ("Normalized Value"=w330:dbl)  [unwired: 8 in, 2 out]
        n203 = call <vilib>:"WPI_PotentiometerGetNormalized.vi"("PotDevRef"=w326) -> ("Normalized Value"=w324:dbl)  [unwired: 8 in, 2 out]
        n204 = call <vilib>:"WPI_PotentiometerGetNormalized.vi"("PotDevRef"=w316) -> ("Normalized Value"=w315:dbl)  [unwired: 8 in, 2 out]
        n205 = call <vilib>:"WPI_PotentiometerGetNormalized.vi"("PotDevRef"=w325) -> ("Normalized Value"=w322:dbl)  [unwired: 8 in, 2 out]
        n206 = Increment(x=w330) -> ()  [unwired: 1 out]
        n207 = Increment(x=w315) -> ()  [unwired: 1 out]
        n208 = Unbundle By Name(w328) -> ("Y-Axis"=w318:dbl)
        n209 = disable-structure shown="Enabled" {
          disable-tunnel: w324 -> [w342 w347]
          disable-tunnel: [w343 w346] -> w323
          disable-tunnel: w320 -> [w341 _]
          frame Enabled {
            n210 = Subtract(x=w342, y=w341) -> (x-y=w345:dbl)
            n211 = Multiply(x=w345, y=-1505.88) -> (x*y=w343:dbl)
          }
          frame Disabled {
            n212 = expression code="-1505.88*(x-.587)"(w347) -> (w346:dbl)
          }
        }
        n213 = disable-structure shown="Enabled" {
          disable-tunnel: w322 -> [w336 w340]
          disable-tunnel: [w334 w339] -> w321
          disable-tunnel: w319 -> [w335 _]
          frame Enabled {
            n214 = Subtract(x=w336, y=w335) -> (x-y=w338:dbl)
            n215 = Multiply(x=w338, y=-1431.77) -> (x*y=w334:dbl)
          }
          frame Disabled {
            n216 = expression code="-1431.77*(x-0.961)"(w340) -> (w339:dbl)
          }
        }
        n217 = Increment(x=w318) -> ()  [unwired: 1 out]
        n218 = call-poly <vilib>:"NT Write Value.vi"("Numeric"=w314, "Name"="Gyro") -> ()  [unwired: 9 in, 1 out]
        n219 = Increment(x=w321) -> ()  [unwired: 1 out]
        n220 = call-poly <vilib>:"NT Write Value.vi"("Numeric"=w323, "Name"="mechanismEncoder") -> ()  [unwired: 9 in, 1 out]
        n221 = Wait (ms)(milliseconds to wait=u32 150) -> ()  [unwired: 1 out]
      }
    }
    frame Disabled {
    }
  }
  n222 = disable-structure shown="Disabled" {
    frame Disabled {
      n223 = call <vilib>:"WPI_RobotDriveRefNum Registry Get.vi"("refnum name"="Drive 1") -> ("RobotDriveDevRef"=w348:T23)  [unwired: 9 in, 1 out]
      n224 = while {
        tunnel: w348 -> [w351]
        stop <- FALSE stop-if-true
        n225 = global read "Robot Global Data.vi" "Porticullis Tele"() -> (w350:bool)
        n226 = case shown="True" w350 {
          tunnel: w351 -> [_ w357]
          frame False {
            # "Nothing :)"
          }
          frame True {
            n227 = call "Set Arm Position.vi"("RobotDriveDevRef 2"=w357, "Setpoint"=100.0) -> ("RobotDriveDevRef"=w356:T23)  [unwired: 9 in]
            n228 = for {
              N: 40 -> [_]
              tunnel: w356 -> [w363]
              tunnel: [w363] -> w355
              n229 = Wait (ms)(milliseconds to wait=u32 50) -> ()  [unwired: 1 out]
            }
            n230 = for {
              N: 60 -> [_]
              tunnel: w355 -> [w361]
              tunnel: [w361] -> _
              n231 = call-poly <vilib>:"WPI_RobotDriveArcadeDrive.vi"("X axis value"=-0.5, "RobotDriveDevRef"=w361) -> ()  [unwired: 7 in, 3 out]
              n232 = Wait (ms)(milliseconds to wait=u32 50) -> ()  [unwired: 1 out]
            }
          }
        }
        n233 = Wait (ms)(milliseconds to wait=u32 200) -> ()  [unwired: 1 out]
      }
    }
    frame Enabled {
    }
  }
  n234 = disable-structure shown="Disabled" {
    frame Disabled {
      n235 = call <vilib>:"WPI_RobotDriveRefNum Registry Get.vi"("refnum name"="Drive 1") -> ("RobotDriveDevRef"=w365:T23)  [unwired: 9 in, 1 out]
      n236 = while {
        tunnel: w365 -> [w368]
        stop <- FALSE stop-if-true
        n237 = global read "Robot Global Data.vi" "CDF Tele"() -> (w367:bool)
        n238 = case shown="True" w367 {
          tunnel: w368 -> [_ w383]
          frame False {
            w371 = FALSE
            # "Nothing :)"
            n239 = global write "Robot Global Data.vi" "Drive Disable"(w371) -> ()
            n240 = global write "Robot Global Data.vi" "Arm Disable"(w371) -> ()
          }
          frame True {
            w374 = TRUE
            n241 = call <vilib>:"WPI_GyroRefNum Registry Get.vi"("refnum name"="Gyro") -> ("GyroDevRef"=w381:T7)  [unwired: 9 in, 1 out]
            n242 = global write "Robot Global Data.vi" "Drive Disable"(w374) -> ()
            n243 = global write "Robot Global Data.vi" "Arm Disable"(w374) -> ()
            n244 = call <vilib>:"WPI_GyroGetAngle.vi"("GyroDevRef"=w381) -> ("Angle"=w379:dbl)  [unwired: 6 in, 4 out]
            n245 = flat-sequence {
              tunnel: [w384] -> w373
              tunnel: w372 -> [_]
              frame #0 {
                n246 = global read "Robot Global Data.vi" "CDF Tele"() -> (w384:bool)
              }
            }
            n247 = call "Forward For inch.vi"("Angle robot facing"=w379, "Speed"=0.65, "Distance"=-13.0, "RobotDriveDevRef in"=w383) -> ("RobotDriveDevRef out"=w372:T23)  [unwired: 7 in]
            n248 = case shown="True" w373 {
              tunnel: w372 -> [w385 w387]
              tunnel: [w385 w386] -> w375
              frame False {
              }
              frame True {
                n249 = call "Set Arm Position.vi"("RobotDriveDevRef 2"=w387, "Speed"=0.9, "Setpoint"=620.0) -> ("RobotDriveDevRef"=w386:T23)  [unwired: 8 in]
                n250 = flat-sequence {
                  tunnel: w386 -> [_]
                  frame #0 {
                    "CDF Arm Down" <- TRUE
                  }
                }
              }
            }
            n251 = while {
              tunnel: w372 -> [w411]
              tunnel: [w410] -> _
              stop <- w406 stop-if-true
              n252 = local read "CDF Arm Down"() -> (w407:bool)
              n253 = global read "Robot Global Data.vi" "CDF Tele"() -> (w405:bool)
              n254 = call-poly <vilib>:"WPI_RobotDriveArcadeDrive.vi"("Y axis value"=-0.35, "X axis value"=0.0 ("Angle robot facing"), "RobotDriveDevRef"=w411) -> ("RobotDriveDevRef"=w410:T23)  [unwired: 6 in, 2 out]
              n255 = Wait (ms)(milliseconds to wait=u32 20) -> ()  [unwired: 1 out]
              n256 = Not(x=w405) -> (.not. x?=w404:bool)
              n257 = Or(x=w407, y=w404) -> (x .or. y?=w406:bool)
            }
            n258 = Tick Count (ms)() -> (millisecond timer value=w377:u32)
            n259 = while {
              tunnel: w375 -> [w402]
              tunnel: [w401] -> w376
              tunnel: w377 -> [w398]
              stop <- w393 stop-if-true
              n260 = global read "Robot Global Data.vi" "CDF Tele"() -> (w395:bool)
              n261 = call "Timeout.vi"("Start Time In"=w398, "Time Limit"=u32 2500) -> ("Timeout"=w394:bool)  [unwired: 8 in, 1 out]
              n262 = Not(x=w395) -> (.not. x?=w396:bool)
              n263 = call-poly <vilib>:"WPI_RobotDriveArcadeDrive.vi"("Y axis value"=-0.65, "X axis value"=0.0 ("Angle robot facing"), "RobotDriveDevRef"=w402) -> ("RobotDriveDevRef"=w401:T23)  [unwired: 6 in, 2 out]
              n264 = Or(x=w394, y=w396) -> (x .or. y?=w393:bool)
              n265 = Wait (ms)(milliseconds to wait=u32 20) -> ()  [unwired: 1 out]
            }
            n266 = while {
              tunnel: w376 -> [_]
              stop <- w391 stop-if-true
              n267 = global read "Robot Global Data.vi" "CDF Tele"() -> (w392:bool)
              n268 = Not(x=w392) -> (.not. x?=w391:bool)
            }
          }
        }
        n269 = Wait (ms)(milliseconds to wait=u32 200) -> ()  [unwired: 1 out]
      }
    }
    frame Enabled {
    }
  }
  n270 = disable-structure shown="Disabled" {
    frame Disabled {
      # "because sometimes the velocity appears to dip to 0 even if the arm is moving, why not add this\nto make sure it is 0 for a period of 100 ms"
      n271 = Less?(y=0.8) -> (x < y?=w416:bool)  [unwired: 1 in]
      n272 = feedback #5(0.0 ("angle B 2")) -> (w415:dbl)
      n273 = case shown="True" w416 {
        tunnel: [0.0 w421] -> w414
        tunnel: w415 -> [_ w420]
        frame False {
        }
        frame True {
          n274 = Increment(x=w420) -> (x+1=w421:dbl)
        }
      }
      n275 = feedback-in #5(w414) -> ()
      n276 = Greater Or Equal?(x=w414, y=5.0) -> ()  [unwired: 1 out]
    }
    frame Enabled {
    }
  }
  n277 = disable-structure shown="Disabled" {
    frame Disabled {
      n278 = while {
        tunnel: i16[] [42, 16464, 3, 6, 16394, 376, 6, 16394, 377, 12, 16417, 1908, 24946, 26469, 29759, 2900, 24946, 26469, 29728, 17505, 29793] ("type string") -> [w423]
        stop <- FALSE stop-if-true
        # "put into PID loop"
        # "Get target information"
        # "if first false\n(target lost)"
        n279 = call-poly <vilib>:"NT Read Value.vi"("Name"="targetData") -> ("error out"=w439:errorcluster, "String"=w436:string)  [unwired: 9 in]
        n280 = Flattened String To Variant(4:w439, 6:w436, 7:w423) -> (0:w437:errorcluster, 3:w438:variant)
        n281 = Variant To Data(error in=w437, type=cluster{"x":dbl, "y":dbl, "target?":bool} {"x"=0.0, "y"=0.0, "target?"=FALSE} ("input cluster"), Variant=w438) -> (data=w432:cluster{"x":dbl, "y":dbl, "target?":bool})  [unwired: 1 out]
        n282 = Unbundle By Name(w432) -> ("target?"=w430:bool)
        n283 = feedback-in #6(w430) -> ()
        n284 = feedback #6(FALSE ("target?")) -> (w429:bool)
        n285 = Less?(x=w430, y=w429) -> (x < y?=w428:bool)
        n286 = feedback #7(cluster{"x out":dbl, "y out":dbl} {"x out"=10000.0, "y out"=0.0}) -> (w425:cluster{"x out":dbl, "y out":dbl})
        n287 = case shown="False" w430 {
          tunnel: w432 -> [_ w488]
          tunnel: [w442 w478] -> w431
          tunnel: w428 -> [w444 _]
          tunnel: [w441 w475] -> w426
          tunnel: w425 -> [w443 _]
          frame False {
            n288 = case shown="False" w444 {
              tunnel: w443 -> [w456 w474]
              tunnel: [w456 w464] -> w441
              tunnel: [w446 w460] -> w442
              frame False {
                # "no target"
                # "Angle to aim = \natan(targetY-robotY/targetX-Robotx)"
                n289 = global read "Robot Global Data.vi" "poses"() -> (w450:cluster{"theta":dbl}[])
                n290 = Index Array(array=w450, index=0) -> (element=w449:cluster{"theta":dbl})
                n291 = Unbundle By Name(w449) -> ("x"=w454:dbl, "y"=w452:dbl)
                n292 = Unbundle(w456) -> ("x out"=w455:dbl, "y out"=w453:dbl)
                n293 = Subtract(x=w455, y=w454) -> (x-y=w447:dbl)
                n294 = Subtract(x=w453, y=w452) -> (x-y=w448:dbl)
                n295 = Inverse Tangent (2 Input)(1:w447, 2:w448) -> (0:w445:dbl)
                n296 = expression code="(x/pi)*180.0" ("radians to degrees")(w445) -> (w446:dbl)
              }
              frame True {
                # "no target"
                # "last target\nlocation"
                # "pose when target last seen"
                # "Find target in field space"
                # "translate by \nrobot location"
                # "rotate by\ngyro angle"
                n297 = global read "Robot Global Data.vi" "poses"() -> (w462:cluster{"theta":dbl}[])
                n298 = Unbundle(w474) -> ("x out"=w458:dbl, "y out"=w457:dbl)
                n299 = Index Array(array=w462, index=19) -> (element=w461:cluster{"theta":dbl})
                n300 = Unbundle(w461) -> (w469:dbl, w468, w467)
                n301 = expression code="(x/180.0)*pi" ("degrees to radians")(w469) -> (w473:dbl)
                n302 = call-poly <vilib>:"2D Cartesian Coordinate Rotation.vi"("theta"=w473, "y"=w457, "x"=w458) -> ("y out"=w471:dbl, "x out"=w472:dbl)  [unwired: 6 in, 1 out]
                n303 = Bundle(w468, w467) -> (w470:cluster{void, void})  [unwired: 1 in]
                n304 = call-poly <vilib>:"2D Cartesian Coordinate Shift.vi"("shift"=w470, "Y"=w471, "X"=w472) -> ("Y Out"=w465:dbl[], "X Out"=w466:dbl[])  [unwired: 6 in, 1 out]
                n305 = Bundle("X Out"=w466, "Y Out"=w465) -> (w464:cluster{"X Out":dbl[], "Y Out":dbl[]})  [unwired: 1 in]
                n306 = Inverse Tangent (2 Input)(1:w458, 2:w457) -> (0:w459:dbl)
                n307 = expression code="(x/pi)*180.0" ("radians to degrees")(w459) -> (w460:dbl)
              }
            }
          }
          frame True {
            # "last seen target"
            # "target visible"
            # "find angle to turn to"
            # "At time picture was taken"
            # "Find angle"
            # "camera offset\n(left + towards rear = positive)"
            n308 = Unbundle By Name(w488) -> ("x"=w487:dbl, "y"=w486:dbl)
            n309 = call-poly <vilib>:"2D Cartesian Coordinate Shift.vi"("shift"=cluster{"dx":dbl, "dy":dbl} {"dx"=0.0, "dy"=0.0}, "y"=w486, "x"=w487) -> ("y out"=w476:dbl, "x out"=w477:dbl)  [unwired: 6 in, 1 out]
            n310 = Inverse Tangent (2 Input)(1:w477, 2:w476) -> (0:w484:dbl)
            n311 = Bundle("x out"=w477, "y out"=w476) -> (w475:cluster{"x out":dbl, "y out":dbl})  [unwired: 1 in]
            n312 = expression code="(x/pi)*180.0" ("radians to degrees")(w484) -> (w483:dbl)
            n313 = global read "Robot Global Data.vi" "poses"() -> (w482:cluster{"theta":dbl}[])
            n314 = Index Array(array=w482, index=19) -> (element=w480:cluster{"theta":dbl})
            n315 = Unbundle By Name(w480) -> ("theta"=w479:dbl)
            n316 = Add(x=w483, y=w479) -> (x+y=w478:dbl)
          }
        }
        n317 = feedback-in #7(w426) -> ()
        n318 = global write "Robot Global Data.vi" "Target Heading"(w431) -> ()
        n319 = Wait (ms)(milliseconds to wait=u32 20) -> ()  [unwired: 1 out]
      }
    }
    frame Enabled {
    }
  }
  n320 = disable-structure shown="Disabled" {
    frame Disabled {
      n321 = while {
        stop <- FALSE stop-if-true
        n322 = global read "Robot Global Data.vi" "Automated Aim"() -> (w490:bool)
        n323 = Wait (ms)(milliseconds to wait=u32 200) -> ()  [unwired: 1 out]
        n324 = case shown="True" w490 {
          frame False {
          }
          frame True {
            n325 = call <vilib>:"WPI_RobotDriveRefNum Registry Get.vi"("refnum name"="Drive 1") -> ("RobotDriveDevRef"=w492:T23)  [unwired: 9 in, 1 out]
            n326 = while {
              tunnel: w492 -> [w496]
              stop <- w500 stop-if-true
              n327 = call-poly <vilib>:"NT Read Value.vi"("Name"="xPosition") -> ("Numeric"=w495:dbl)  [unwired: 9 in, 1 out]
              n328 = Subtract(x=w495, y=85.0) -> (x-y=w505:dbl)
              n329 = Not Equal To 0?(x=w495) -> (x != 0?=w494:bool)
              n330 = Divide(x=w505, y=80.0) -> (x/y=w503:dbl)
              n331 = call-poly <vilib>:"PID.vi"("output range"=cluster{"output high":dbl, "output low":dbl} {"output high"=0.6, "output low"=-0.6}, "PID gains"=T10 {"proportional gain (Kc)"=5.0, "integral time (Ti, min)"=0.03, "derivative time (Td, min)"=0.03} ("Turn robot to camera 2"), "process variable"=w503, "setpoint"=0.0) -> ("output"=w509:dbl)  [unwired: 6 in, 1 out]
              n332 = global read "Robot Global Data.vi" "Automated Aim"() -> (w501:bool)
              n333 = Negate(x=w509) -> (-x=w499:dbl)
              n334 = Select(t=w499, s=w494, f=0.0) -> (s? t:f=w497:dbl)
              n335 = Wait (ms)(milliseconds to wait=u32 20) -> ()  [unwired: 1 out]
              n336 = call-poly <vilib>:"WPI_RobotDriveArcadeDrive.vi"("X axis value"=w497, "RobotDriveDevRef"=w496) -> ()  [unwired: 7 in, 3 out]
              n337 = Not(x=w501) -> (.not. x?=w500:bool)
            }
          }
        }
      }
    }
    frame Enabled {
    }
  }
  n338 = disable-structure shown="Disabled" {
    frame Disabled {
      n339 = for {
        N: 4 -> [_]
        n340 = for {
          N: 3 -> [_]
          tunnel: _ -> [w517]
          tunnel: [w518] -> w515
          n341 = call <vilib>:"WPI_MotorControlSetOutput.vi"("Output"=-0.35 ("Left axis value"), "MotorControlDevRef"=w517) -> ("MotorControlDevRef"=w518:T11)  [unwired: 7 in, 2 out]
          n342 = Wait (ms)(milliseconds to wait=u32 50) -> ()  [unwired: 1 out]
        }
        n343 = for {
          N: 3 -> [_]
          tunnel: w515 -> [w521]
          tunnel: [w522] -> _
          n344 = call <vilib>:"WPI_MotorControlSetOutput.vi"("Output"=0.35 ("Left axis value"), "MotorControlDevRef"=w521) -> ("MotorControlDevRef"=w522:T11)  [unwired: 7 in, 2 out]
          n345 = Wait (ms)(milliseconds to wait=u32 50) -> ()  [unwired: 1 out]
        }
      }
    }
    frame Enabled {
    }
  }
  n346 = disable-structure shown="Enabled" {
    frame Enabled {
      n347 = Random Number (0-1)() -> (number: 0 to 1=w527:dbl)
      n348 = Format Into String(format string="/home/lvuser/data-%.6f.csv", w527) -> (resulting string=w525:string)  [unwired: 2 in, 1 out]
      n349 = String To Path(string=w525) -> (path=w524:path)
      n350 = Open/Create/Replace File(file path (use dialog)=w524, operation (0:open)=T24."replace or create", access (0:read/write)=enum16{"read/write", "read-only", "write-only"}."write-only") -> (refnum out=w532:refnum<file>, error out=w529:errorcluster)  [unwired: 3 in, 1 out]
      n351 = while {
        tunnel: w532 -> [w556]
        tunnel: [w543] -> w531
        tunnel: w529 -> [w538]
        tunnel: [w534] -> w528
        i -> [w554]
        stop <- FALSE stop-if-true
        w555 = u32 50 ("milliseconds to wait")
        # "This while loop can be used \nif other data needs to be written. \nDisabled for now because we don't need to write \nany other data."
        n352 = Wait (ms)(milliseconds to wait=w555) -> ()  [unwired: 1 out]
        n353 = Multiply(x=w555, y=w554) -> (x*y=w553:u32)
        n354 = call <vilib>:"WPI_Power Get PDP Currents.vi"() -> ("all currents (A)"=w542:dbl[])  [unwired: 13 in, 2 out]
        n355 = call <vilib>:"WPI_Power Get PDP Voltage.vi"() -> ("voltage (V)"=w547:dbl)  [unwired: 14 in, 1 out]
        n356 = Number To Decimal String(number=w553) -> (decimal integer string=w552:string)  [unwired: 1 in]
        n357 = Write to Text File(file (use dialog)=w556, text=w552, error in=w538) -> (refnum out=w551:refnum<file>, error out=w537:errorcluster)  [unwired: 1 in, 1 out]
        n358 = Write to Text File(file (use dialog)=w551, text=",", error in=w537) -> (refnum out=w550:refnum<file>, error out=w536:errorcluster)  [unwired: 1 in, 1 out]
        n359 = Build Array (concatenate)(w542, w547) -> (w546:dbl[])
        n360 = for {
          tunnel: w550 -> [w570]
          tunnel: [w564] -> w548
          tunnel: w546 -> [w563] mode=indexing
          tunnel: w536 -> [w562]
          tunnel: [w561] -> w535
          n361 = Format Into String(format string="%f", w563) -> (resulting string=w568:string)  [unwired: 2 in, 1 out]
          n362 = Write to Text File(file (use dialog)=w570, text=w568, error in=w562) -> (refnum out=w566:refnum<file>, error out=w567:errorcluster)  [unwired: 1 in, 1 out]
          n363 = Write to Text File(file (use dialog)=w566, text=",", error in=w567) -> (refnum out=w564:refnum<file>, error out=w561:errorcluster)  [unwired: 1 in, 1 out]
        }
        n364 = disable-structure shown="Enabled" {
          disable-tunnel: w548 -> [w559 w560]
          disable-tunnel: [w557 w560] -> w544
          frame Disabled {
            n365 = for {
              n366 = Write to Text File() -> ()  [unwired: 4 in, 3 out]
            }
            n367 = Write to Text File(file (use dialog)=w559, text="\n") -> (refnum out=w557:refnum<file>)  [unwired: 2 in, 2 out]
          }
          frame Enabled {
          }
        }
        n368 = Concatenate Strings("\r", "\n") -> (w539:string)
        n369 = Write to Text File(file (use dialog)=w544, text=w539, error in=w535) -> (refnum out=w543:refnum<file>, error out=w534:errorcluster)  [unwired: 1 in, 1 out]
      }
      n370 = Close File(refnum=w531, error in=w528) -> ()  [unwired: 2 out]
    }
    frame Disabled {
    }
  }
  "error out (no error)" <- "error in (no error)"
